vi "Pigeon Gyro.vi"(0 "Reset Yaw?":bool) -> (1 "YPR.Yaw":dbl, 2 "YPR.Yaw Rate":dbl)   [LabVIEW 2016, in "Apple script.lvlib"]
uses:
  Apple script.lvlib
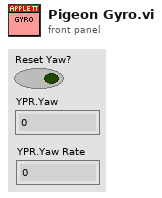
[diagram p1: front panel]
types:
  T1 = typedef "CTRE_PigeonIMU_DeviceRef.ctl" = cluster{"DeviceStatus":errorcluster, "Device Number":u8, "Type":T2, "Device ID":u32}
  T2 = typedef "CTRE_PigeonIMU_ConnectionType.ctl" = u32
  T3 = typedef "CTRE_PigeonIMU_GlobalStatus.ctl" = cluster{"PigeonState":T4, "FusedHeading":cluster{"Heading":dbl, "Valid?":bool, "Fusing?":bool}, "YPR":cluster{"Yaw":dbl, "Pitch":dbl, "Roll":dbl}, "Compass":cluster{"Heading":dbl, "Magnitude":dbl, "Absolute Heading":dbl}, "Accelerometer":cluster{"Biased":cluster{"X":i16, "Y":i16, "Z":i16, "Norm":i16}, "Angles":cluster{"XZ Tilt":dbl, "YZ Tilt":dbl, "XY Tilt":dbl}}, "Magnetometer":cluster{"Raw":cluster{"X":i16, "Y":i16, "Z":i16}, "Biased":cluster{"X":i16, "Y":i16, "Z":i16}}, "Gyro":cluster{"X":dbl, "Y":dbl, "Z":dbl, "Norm":dbl}, "6D Quaternian":cluster{"W":dbl, "X":dbl, "Y":dbl, "Z":dbl}, "Temp. (C)":dbl, "UpTime":u32, "StartupStatus":cluster{"ResetCount":i32, "ResetFlags":i32, "FirmwareVersion":i32, "HasReset?":bool}, "Calibration":cluster{"CurrentMode":T5, "LastCalError":i32, "CalBooting?":bool}, "CAN Error":errorcluster, "AccumGyro":cluster{"X":dbl, "Y":dbl, "Z":dbl}, "Usage Frame":u32}
  T4 = typedef "CTRE_PigeonIMU_PigeonState.ctl" = enum16{"NoComm", "Initializing", "Ready", "UserCalibration"}
  T5 = typedef "CTRE_PigeonIMU_CalibrationMode.ctl" = u16
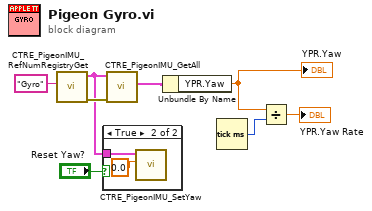
[diagram p0: block diagram]
diagram:
  n1 = call <vilib>:"CTRE_PigeonIMU_RefNumRegistryGet.vi"("refnum name"="Gyro") -> ("error out"=w8:errorcluster, "PigeonIMUDevRef"=w6:T1)  [unwired: 9 in]
  n2 = case shown="True" "Reset Yaw?" {
    tunnel: w6 -> [_ w10]
    frame False {
    }
    frame True {
      n3 = call <vilib>:"CTRE_PigeonIMU_SetYaw.vi"("Value"=0.0, "PigeonIMUDevRef"=w10) -> ()  [unwired: 8 in, 2 out]
    }
  }
  n4 = call <vilib>:"CTRE_PigeonIMU_GetAll.vi"("error in (no error)"=w8, "PigeonIMUDevRef"=w6) -> ("Get All"=w7:T3)  [unwired: 7 in, 2 out]
  n5 = Unbundle By Name(w7) -> ("YPR.Yaw"=w2:dbl)
  "YPR.Yaw" <- w2
  n6 = Tick Count (ms)() -> (millisecond timer value=w3:u32)
  n7 = Divide(x=w2, y=w3) -> (x/y=→"YPR.Yaw Rate":dbl)
